vi "Get Home Mode from Config.vi"(8 "error in (no error)":errorcluster) -> (0 "error out":errorcluster, 3 "Home Mode":i32)   [LabVIEW 2020, in "ESP301.lvlib"]
uses:
  ESP301.lvlib
  <vilib>/Utility/config.llb/Read Key (I32).vi
  <vilib>/Utility/config.llb/NI_LVConfig.lvlib
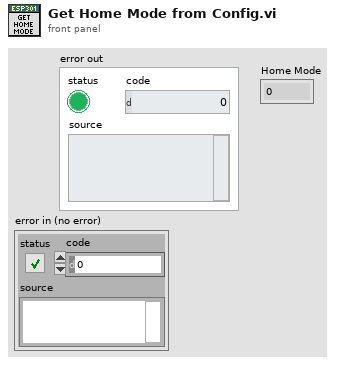
[diagram p1: front panel]
types:
  T1 = typedef "NI_LVConfig.lvlib/Config Data RefNum.ctl" = refnum<k1>
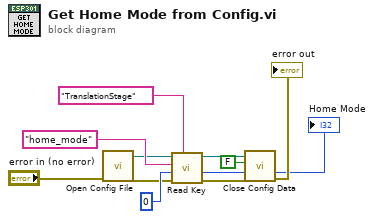
[diagram p0: block diagram]
diagram:
  n1 = call "Open Config File.vi"("error in (no error)"="error in (no error)") -> ("error out"=w3:errorcluster, "Refnum out"=w4:T1)  [unwired: 9 in]
  n2 = call-poly <vilib>:"Read Key.vi"("section"="TranslationStage", "error in (no error)"=w3, "default value"=0, "key"="home_mode", "refnum"=w4) -> ("error out"=w8:errorcluster, "value"=→"Home Mode":i32, "refnum out"=w9:T1)  [unwired: 3 in, 1 out]
  n3 = call <vilib>:"Close Config Data.vi"("error in (no error)"=w8, "write file if changed (T)"=FALSE, "refnum"=w9) -> ("error out"=→"error out":errorcluster)  [unwired: 7 in, 1 out]
